vi "Write RunTimeObjectType.vi"(8 "error in (no error)":errorcluster, 10 "RunTimeObjectType":T1, 11 "RunTimeObjectsSection in":refnum<class "RunTimeObjectsSection.lvclass">) -> (0 "error out":errorcluster, 3 "RunTimeObjectsSection out":refnum<class "RunTimeObjectsSection.lvclass">)   [LabVIEW 2015, in "RunTimeObjectsSection.lvclass"]
uses:
  RunTimeObjectsSection.lvclass
  Custom Device Type Defs/RunTimeObjectTypes.ctl
  RunTimeObjectsSection.lvclass/RunTimeObjectsSection.ctl
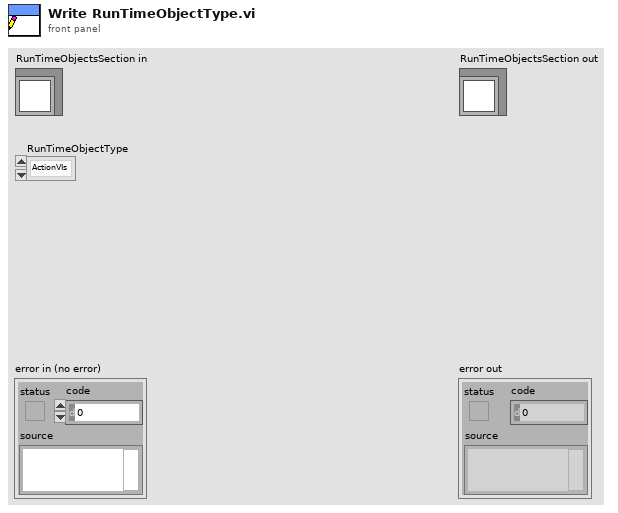
[diagram p1: front panel]
types:
  T1 = typedef "RunTimeObjectTypes.ctl" = enum16{"ActionVIs", "ButtonList", "RunTimeMenu"}
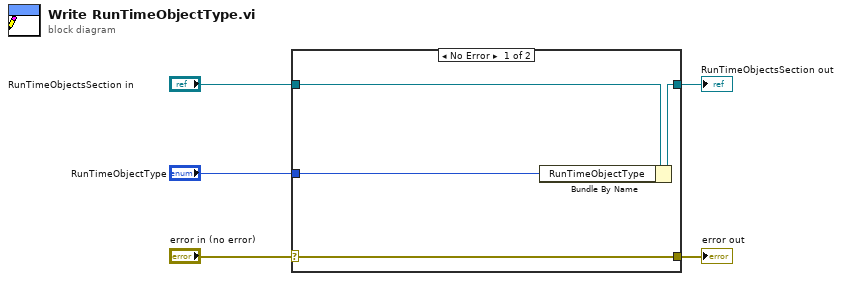
[diagram p0: block diagram]
diagram:
  n1 = case shown="No Error" "error in (no error)" {
    selector: "error in (no error)" -> [w9 w10]
    tunnel: [w9 w10] -> w4
    tunnel: [w7 w11] -> w2
    tunnel: "RunTimeObjectsSection in" -> [w8 w11]
    tunnel: "RunTimeObjectType" -> [w6 _]
    frame No Error {
      n2 = Bundle By Name(cluster=w8, "RunTimeObjectType"=w6) -> (w7:refnum<class "RunTimeObjectsSection.lvclass">)
    }
    frame Error {
    }
  }
  "error out" <- w4
  "RunTimeObjectsSection out" <- w2
